vi "oa_Front Extrapolation Processing.vi"(9 "pulse history in [s]":dbl[](array[numeric]) format="%.2f", 11 "pulse positions in [s]":dbl[](array[numeric]) format="%.2f") -> (1 "pulse history out [s]":dbl[](array[numeric]) format="%.2f", 2 "pulse new history out [s]":dbl[](array[numeric]) format="%.2f", 3 "pulse positions out [s]":dbl[](array[numeric]) format="%.2f")   [LabVIEW 2017, in "SoundVib_TachProcess.lvlib"]
uses:
  <vilib>/addons/Sound and Vibration/Order Analysis/Tach Process/SoundVib_TachProcess.lvlib
  <vilib>/Analysis/1siggen.llb/Ramp Pattern by Samples.vi
  <vilib>/Analysis/NI_AALPro.lvlib
  <vilib>/Analysis/NI_AALBase.lvlib
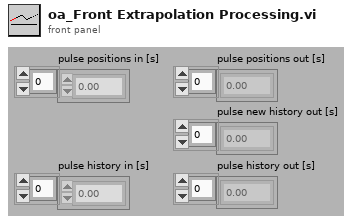
[diagram p1: front panel]
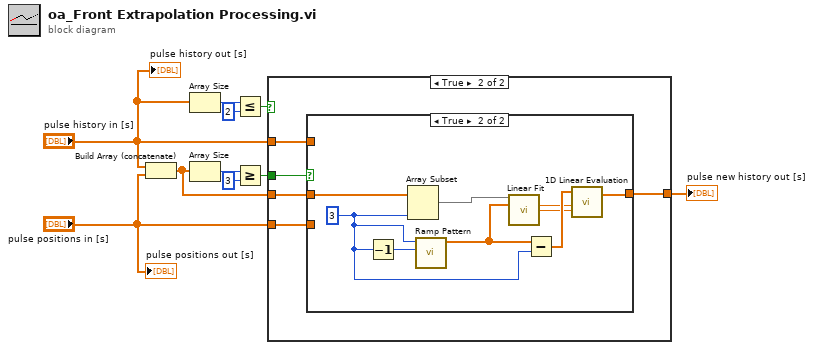
[diagram p0: block diagram]
diagram:
  n1 = Build Array (concatenate)("pulse history in [s]", "pulse positions in [s]") -> (w5:dbl[])
  n2 = Array Size(array="pulse history in [s]") -> (size(s)=w10:i32)
  n3 = Array Size(array=w5) -> (size(s)=w8:i32)
  n4 = Less Or Equal?(x=w10, y=2) -> (x <= y?=w3:bool)
  n5 = Greater Or Equal?(x=w8, y=3) -> (x >= y?=w4:bool)
  n6 = case shown="True" w3 {
    tunnel: "pulse history in [s]" -> [_ w15]
    tunnel: [_ w14] -> w6
    tunnel: w5 -> [_ w13]
    tunnel: "pulse positions in [s]" -> [_ w12]
    tunnel: w4 -> [_ w11]
    frame False {
    }
    frame True {
      n7 = case shown="True" w11 {
        tunnel: w15 -> [_ _]
        tunnel: [_ w21] -> w14
        tunnel: w13 -> [_ w19]
        tunnel: w12 -> [_ _]
        frame False {
        }
        frame True {
          w18 = 3 ("extrapolation length")
          n8 = Decrement(x=w18) -> (x-1=w16:i32)
          n9 = Array Subset(array=w19, length=w18) -> (w20:dbl[])  [unwired: 1 in]
          n10 = call-poly <vilib>:"Ramp Pattern.vi"("end"=w16, "samples"=w18) -> ("Ramp Pattern"=w17:dbl[])  [unwired: 8 in, 1 out]
          n11 = call <vilib>:"Linear Fit.vi"("Y"=w20, "X"=w17) -> ("slope"=w23:dbl, "intercept"=w22:dbl)  [unwired: 9 in, 3 out]
          n12 = Subtract(x=w17, y=w18) -> (x-y=w24:dbl[])
          n13 = call <vilib>:"1D Linear Evaluation.vi"("offset"=w22, "scale"=w23, "X"=w24) -> ("Y[i]=X[i]*a+b"=w21:dbl[])  [unwired: 1 out]
        }
      }
    }
  }
  "pulse new history out [s]" <- w6
  "pulse positions out [s]" <- "pulse positions in [s]"
  "pulse history out [s]" <- "pulse history in [s]"
